vi "STSGrid.vi"(9 "Settings":T1={"Cutoff frq I/V"=0.125, "Cutoff frq dI/dV"=0.125, "Filter order dI/DV"=2, "Filter type  dI/dV"=enum."Gaussian", "Filter order I/V"=2, "Filter type I/V"=enum."Gaussian"} {"Filter order I/V" min=1 max=1000 step=1; "Filter order dI/DV" min=1 max=1000 step=1}, 11 "Binary Spectroscopy File":path) -> ()   [LabVIEW 2014]
uses:
  <userlib>/Nanonis Prog Interface V5/Nanonis Prog Interface.lvlib
panel:
  out "error out Write file":errorcluster
  out "error out Read file":errorcluster
  out "Progress":u8(slide) scale=0.0..100.0
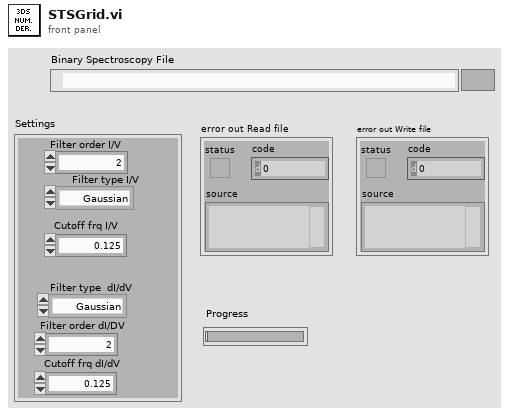
[diagram p1: front panel]
types:
  T1 = cluster{"Cutoff frq I/V":dbl, "Cutoff frq dI/dV":dbl, "Filter order dI/DV":i32, "Filter type  dI/dV":enum16{"none", "Gaussian", "Butterworth", "5th order FIR"}, "Filter order I/V":i32, "Filter type I/V":enum16{"none", "Gaussian", "Butterworth", "5th order FIR"}}
  T2 = typedef "Nanonis Prog Interface.lvlib/Binary_SpectroscopyFile-Config.ctl" = cluster{"Num Par":i32, "Exp size":i32, "Points":i32, "Grid Dim X":i32, "Grid Dim Y":i32, "Header size":i32, "Channels":string[], "Parameters":string[], "Sweep Signal":string, "Grid":cluster{"center X (m)":sgl, "center Y (m)":sgl, "width (m)":sgl, "height (m)":sgl, "angle (deg)":sgl}}
  T3 = cluster{"center X (m)":sgl, "center Y (m)":sgl, "width (m)":sgl, "height (m)":sgl, "angle (deg)":sgl}
  T4 = enum16{"none", "Gaussian", "Butterworth", "5th order FIR"}
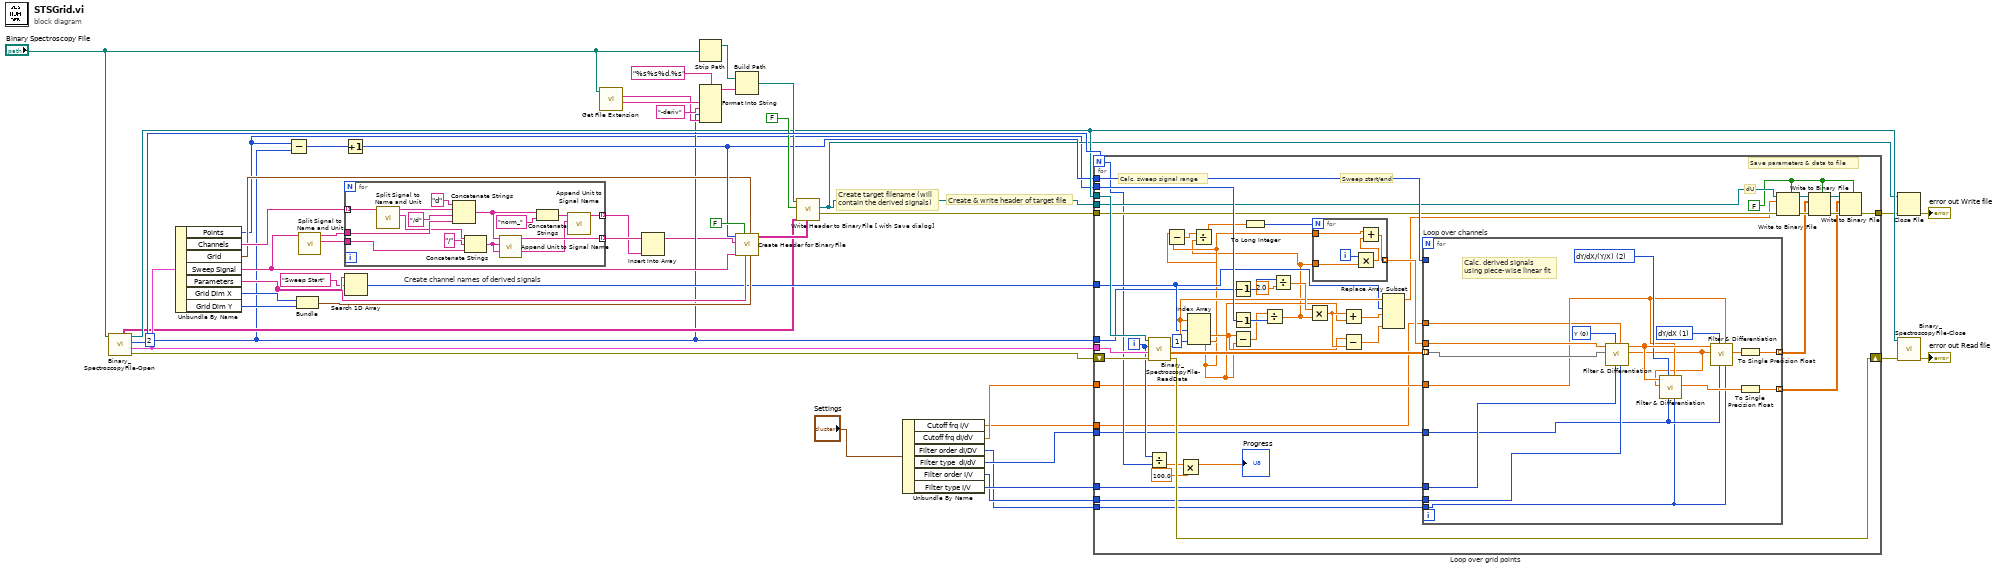
[diagram p0: block diagram]
diagram:
  w12 = u16 2 ("Fit length for derivative")
  # "Create & write header of target file"
  # "Create target filename (will contain the derived signals)"
  n1 = call <userlib>:"Binary_SpectroscopyFile-Open.vi"("Binary Spectroscopy File"="Binary Spectroscopy File") -> ("error out"=w46:errorcluster, "Config"=w34:T2, "Number of Experiments"=w47:i32, "File ref"=w35:refnum<file>, "Global Attributes"=w18:string[][])  [unwired: 6 in]
  n2 = Unbundle By Name(w34) -> ("Points"=w8:i32, "Channels"=w33:string[], "Grid"=w24:T3, "Sweep Signal"=w32:string, "Parameters"=w28:string[], "Grid Dim X"=w44:i32, "Grid Dim Y"=w43:i32)
  n3 = Subtract(x=w8, y=w12) -> (x-y=w29:i32)
  n4 = Bundle("Grid Dim X"=w44, "Grid Dim Y"=w43) -> (w42:cluster{"Grid Dim X":i32, "Grid Dim Y":i32})  [unwired: 1 in]
  n5 = call <userlib>:"Split Signal to Name and Unit.vi"("Name with unit"=w32) -> ("Unit"=w30:string, "Name"=w31:string)  [unwired: 5 in]
  n6 = Increment(x=w29) -> (x+1=w25:i32)
  n7 = for "Create channel names of derived signals" {
    tunnel: w33 -> [w61] mode=indexing
    tunnel: w31 -> [w57]
    tunnel: w30 -> [w54]
    tunnel: [w53] -> w10 mode=indexing
    tunnel: [w48] -> w9 mode=indexing
    n8 = call <userlib>:"Split Signal to Name and Unit.vi"("Name with unit"=w61) -> ("Unit"=w56:string, "Name"=w60:string)  [unwired: 5 in]
    n9 = Concatenate Strings("d" ("string"), w60, "/d" ("string"), w57) -> (w51:string)
    n10 = Concatenate Strings(w56, "/" ("string"), w54) -> (w52:string)
    n11 = call <userlib>:"Append Unit to Signal Name.vi"("Unit"=w52, "Name"=w51) -> ("Name with unit"=w53:string)  [unwired: 5 in]
    n12 = Concatenate Strings(w51, "norm_" ("string")) -> (w50:string)
    n13 = call <userlib>:"Append Unit to Signal Name.vi"("Unit"=w52, "Name"=w50) -> ("Name with unit"=w48:string)  [unwired: 5 in]
  }
  n14 = Search 1D Array(1D array=w28, element="Sweep Start") -> (index of element=w26:i32)  [unwired: 1 in]
  n15 = call <vilib>:"Get File Extension.vi"("file"="Binary Spectroscopy File") -> ("filename without extension"=w15:string, "lowercase file extension"=w14:string)  [unwired: 7 in, 2 out]
  n16 = Insert Into Array(array=w10, new element=w9) -> (w11:string[])  [unwired: 1 in]
  n17 = Strip Path(path="Binary Spectroscopy File") -> (stripped path=w40:path)  [unwired: 1 out]
  n18 = Format Into String(format string="%s%s%d.%s", w15, "-deriv" ("string"), w12, w14) -> (resulting string=w13:string)  [unwired: 2 in, 1 out]
  n19 = Build Path(base path=w40, name or relative path=w13) -> (appended path=w39:path)
  n20 = call <userlib>:"Create Header for BinaryFile.vi"("Grid points"=w42, "Grid param"=w24, "Fixed parameters"=w28, "Backward sweep"=FALSE, "Sweep signal"=w32, "Channels"=w11, "Points per sweep"=w25) -> ("Header (fixed attributes)"=w37:string[][])  [unwired: 4 in]
  n21 = call <userlib>:"Write Header to BinaryFile [ with Save dialog].vi"("Fixed Attributes"=w37, "Attributes in"=w18, "Show Dialog? (T)"=FALSE, "Filename"=w39) -> ("Error out"=w23:errorcluster, "File ref"=w21:refnum<file>)  [unwired: 4 in, 2 out]
  n22 = Unbundle By Name("Settings") -> ("Cutoff frq I/V"=w5:dbl, "Cutoff frq dI/dV"=w6:dbl, "Filter order dI/DV"=w1:i32, "Filter type  dI/dV"=w2:T4, "Filter order I/V"=w3:i32, "Filter type I/V"=w4:T4)
  n23 = for "Loop over grid points" {
    N: w47 -> [w70]
    tunnel: w35 -> [w110]
    tunnel: w34 -> [w109]
    shift-right: [w107] -> w36
    shift-left: w46 -> [w108]
    tunnel: w21 -> [w93]
    tunnel: w12 -> [w82]
    tunnel: w26 -> [w98]
    tunnel: w8 -> [w106]
    tunnel: w25 -> [w95]
    tunnel: w23 -> [w92]
    tunnel: [w89] -> w22
    tunnel: w6 -> [w67]
    tunnel: w5 -> [w66]
    tunnel: w4 -> [w65]
    tunnel: w3 -> [w64]
    tunnel: w2 -> [w63]
    tunnel: w1 -> [w62]
    i -> [w71]
    w86 = FALSE ("prepend array or string size? (T)")
    # "dU"
    # "Sweep start/end"
    # "Save parameters & data to file"
    # "Calc. sweep signal range"
    n24 = call <userlib>:"Binary_SpectroscopyFile-ReadData.vi"("error in"=w108, "Config"=w109, "Experiment to read (Index)"=w71, "File ref In"=w110) -> ("error out"=w107:errorcluster, "data"=w84:sgl[][], "Parameter values"=w99:sgl[])  [unwired: 4 in, 1 out]
    n25 = Divide(x=w71, y=w70) -> (x/y=w72:dbl)
    n26 = Multiply(x=w72, y=100.0) -> (x*y=→"Progress":dbl)
    n27 = Index Array(array=w99, index #1=w98, index #3=1 ("index")) -> (element #1=w77:sgl, element #2=w80:sgl, element #3=w78:sgl)  [unwired: 1 in]
    n28 = Subtract(x=w78, y=w77) -> (x-y=w76:sgl)
    n29 = Decrement(x=w82) -> (x-1=w103:u16)
    n30 = Decrement(x=w106) -> (x-1=w105:i32)
    n31 = Subtract(x=w80, y=w77) -> (x-y=w104:sgl)
    n32 = Divide(x=w104, y=w105) -> (x/y=w75:sgl)
    n33 = Divide(x=w76, y=w75) -> (x/y=w74:sgl)
    n34 = To Long Integer(number=w74) -> (32bit integer=w73:i32)
    n35 = Divide(x=w103, y=sgl 2.0) -> (x/y=w101:sgl)
    n36 = Multiply(x=w101, y=w75) -> (x*y=w100:sgl)
    n37 = for {
      N: w73 -> [_]
      tunnel: w75 -> [w114]
      tunnel: [w112] -> w94 mode=indexing
      tunnel: w77 -> [w111]
      i -> [w115]
      n38 = Multiply(x=w115, y=w114) -> (x*y=w113:sgl)
      n39 = Add(x=w111, y=w113) -> (x+y=w112:sgl)
    }
    n40 = Add(x=w100, y=w77) -> (x+y=w97:sgl)
    n41 = Subtract(x=w80, y=w100) -> (x-y=w96:sgl)
    n42 = Replace Array Subset(array=w99, new element #1=w97, index #1=w98, new element #2=w96) -> (w81:sgl[])  [unwired: 1 in]
    n43 = for "Loop over channels" {
      tunnel: w84 -> [w124] mode=indexing
      tunnel: w95 -> [_]
      tunnel: w94 -> [w132]
      tunnel: [w131] -> w87 mode=indexing
      tunnel: [w130] -> w83 mode=indexing
      tunnel: w67 -> [w123]
      tunnel: w66 -> [w122]
      tunnel: w65 -> [w121]
      tunnel: w64 -> [w120]
      tunnel: w63 -> [w119]
      tunnel: w62 -> [w118]
      w125 = u16 2 items=["Y", "dY/dX", "dY/dX/(Y/X)"] ("Display (Y)")
      w128 = u16 1 items=["Y", "dY/dX", "dY/dX/(Y/X)"] ("Display (Y)")
      w129 = u16 0 items=["Y", "dY/dX", "dY/dX/(Y/X)"] ("Display (Y)")
      # "Calc. derived signals using piece-wise linear fit"
      n44 = call <userlib>:"Filter & Differentiation.vi"("Filter order (2)"=w120, "Cutoff frq (0.125)"=w122, "Filter type (none)"=w121, "Display (Y)"=w129, "Y in"=w124, "X in"=w132) -> ("Y out"=w116:dbl[], "X out"=w127:dbl[])  [unwired: 3 in, 1 out]
      n45 = call <userlib>:"Filter & Differentiation.vi"("Filter order (2)"=w118, "Cutoff frq (0.125)"=w123, "Filter type (none)"=w119, "Display (Y)"=w125, "Y in"=w116, "X in"=w127) -> ("Y out"=w126:dbl[])  [unwired: 3 in, 2 out]
      n46 = call <userlib>:"Filter & Differentiation.vi"("Filter order (2)"=w118, "Cutoff frq (0.125)"=w123, "Filter type (none)"=w119, "Display (Y)"=w128, "Y in"=w116, "X in"=w127) -> ("Y out"=w117:dbl[])  [unwired: 3 in, 2 out]
      n47 = To Single Precision Float(number=w117) -> (single precision float=w131:sgl[])
      n48 = To Single Precision Float(number=w126) -> (single precision float=w130:sgl[])
    }
    n49 = Write to Binary File(file (use dialog)=w93, data=w81, error in=w92, 5:w86) -> (refnum out=w91:refnum<file>, error out=w90:errorcluster)  [unwired: 2 in, 1 out]
    n50 = Write to Binary File(file (use dialog)=w91, data=w87, error in=w90, 5:w86) -> (refnum out=w85:refnum<file>, error out=w88:errorcluster)  [unwired: 2 in, 1 out]
    n51 = Write to Binary File(file (use dialog)=w85, data=w83, error in=w88, 5:w86) -> (error out=w89:errorcluster)  [unwired: 2 in, 2 out]
  }
  n52 = Close File(refnum=w21, error in=w22) -> (error out=→"error out Write file":errorcluster)  [unwired: 1 out]
  n53 = call <userlib>:"Binary_SpectroscopyFile-Close.vi"("error in"=w36, "File ref"=w35) -> ("error out"=→"error out Read file":errorcluster)  [unwired: 9 in]
